vi "UpdateGraphs.vi"(8 "Show buffers":bool, 9 "Buffer mode":T1, 10 "Display mode":T2, 11 "Graph_refs":T3) -> ()   [LabVIEW 2018]
uses:
  controls/Graph_references.ctl
  controls/graph_controls.ctl
  controls/Data_calc_mode.ctl
  controls/Data_display_mode.ctl
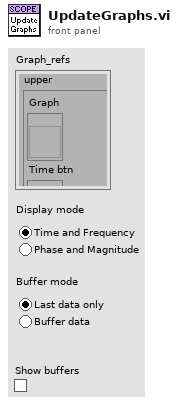
[diagram p1: front panel]
types:
  T1 = typedef "Data_display_mode.ctl" = enum32{"Last data only", "Buffer data"}
  T2 = typedef "Data_calc_mode.ctl" = enum32{"Time and Frequency", "Phase and Magnitude"}
  T3 = typedef "Graph_references.ctl" = cluster{"upper":T4, "lower":T4, "Freq graph":refnum<vi>, "Adaptive FF graph":refnum<vi>}
  T4 = typedef "graph_controls.ctl" = cluster{"Graph":refnum<vi>, "Time btn":refnum<vi>, "Amplitude btn":refnum<vi>, "Chart":refnum<vi>}
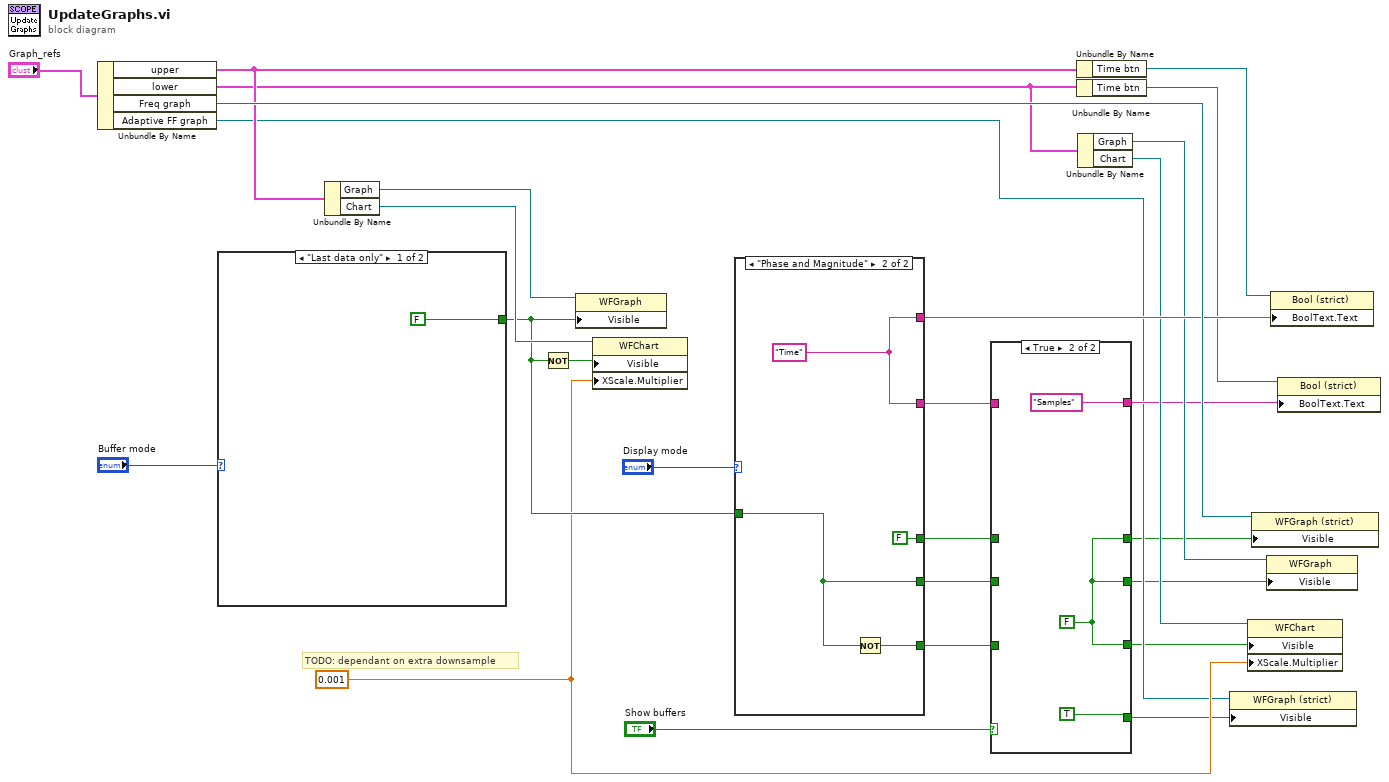
[diagram p0: block diagram]
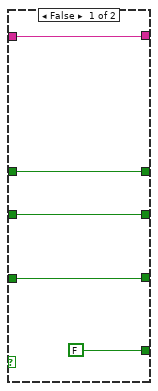
[diagram p2: hidden frame]
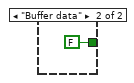
[diagram p3: hidden frame]
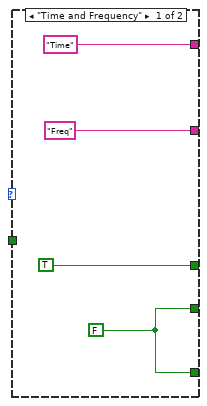
[diagram p4: hidden frame]
diagram:
  w12 = 0.001 ("X Scale.Offset and Multiplier:Multiplier")
  # "TODO: dependant on extra downsample"
  n1 = Unbundle By Name("Graph_refs") -> ("upper"=w20:T4, "lower"=w16:T4, "Freq graph"=w23:refnum<vi>, "Adaptive FF graph"=w9:refnum<vi>)
  n2 = case shown="\"Last data only\"" "Buffer mode" {
    tunnel: [FALSE FALSE] -> w15
    frame "Last data only" {
    }
    frame "Buffer data" {
    }
  }
  n3 = Unbundle By Name(w20) -> ("Graph"=w19:refnum<vi>, "Chart"=w18:refnum<vi>)
  n4 = Not(x=w15) -> (.not. x?=w17:bool)
  n5 = property class="WFGraph"(reference=w19, "Visible"=w15) -> ()  [unwired: 1 in, 2 out]
  n6 = property class="WFChart"(reference=w18, "Visible"=w17, "XScale.Multiplier"=w12) -> ()  [unwired: 1 in, 2 out]
  n7 = case shown="\"Phase and Magnitude\"" "Display mode" {
    tunnel: [TRUE FALSE] -> w2
    tunnel: ["Time" ("Boolean Text.Text") w37] -> w22
    tunnel: ["Freq" ("Boolean Text.Text") w37] -> w11
    tunnel: w15 -> [_ w35]
    tunnel: [w30 w35] -> w4
    tunnel: [w30 w34] -> w7
    frame "Time and Frequency" {
      w30 = FALSE
    }
    frame "Phase and Magnitude" {
      w37 = "Time" ("Boolean Text.Text")
      n8 = Not(x=w35) -> (.not. x?=w34:bool)
    }
  }
  n9 = case shown="True" "Show buffers" {
    tunnel: w11 -> [w42 _]
    tunnel: [w42 "Samples"] -> w10
    tunnel: [FALSE TRUE] -> w8
    tunnel: [w40 w43] -> w6
    tunnel: w7 -> [w40 _]
    tunnel: [w39 w43] -> w5
    tunnel: w4 -> [w39 _]
    tunnel: [w38 w43] -> w3
    tunnel: w2 -> [w38 _]
    frame False {
    }
    frame True {
      w43 = FALSE
    }
  }
  n10 = Unbundle By Name(w20) -> ("Time btn"=w24:refnum<vi>)
  n11 = Unbundle By Name(w16) -> ("Time btn"=w21:refnum<vi>)
  n12 = Unbundle By Name(w16) -> ("Graph"=w13:refnum<vi>, "Chart"=w14:refnum<vi>)
  n13 = property class="WFGraph (strict)"(reference=w9, "Visible"=w8) -> ()  [unwired: 1 in, 2 out]
  n14 = property class="WFChart"(reference=w14, "Visible"=w6, "XScale.Multiplier"=w12) -> ()  [unwired: 1 in, 2 out]
  n15 = property class="WFGraph (strict)"(reference=w23, "Visible"=w3) -> ()  [unwired: 1 in, 2 out]
  n16 = property class="WFGraph"(reference=w13, "Visible"=w5) -> ()  [unwired: 1 in, 2 out]
  n17 = property class="Bool (strict)"(reference=w24, "BoolText.Text"=w22) -> ()  [unwired: 1 in, 2 out]
  n18 = property class="Bool (strict)"(reference=w21, "BoolText.Text"=w10) -> ()  [unwired: 1 in, 2 out]
